vi "SRDG535.PC Set Output.vi"(0 "i ref in":refnum<vi>, 1 "inversion":bool, 2 "amplitude":dbl=1.0 min=-3.0 max=4.0 format="%.2f", 3 "offset":dbl min=-3.0 max=4.0 format="%.2f", 4 "output":u16(ring) items=["T0", "A", "B", "AB", "C", "D", "CD"], 5 "error IO":errorcluster, 7 "mode":i32(ring) items=["TTL", "NIM", "ECL", "VAR"], 9 "load":bool) -> (14 "i ref out":refnum<vi>, 19 "error out":errorcluster)   [LabVIEW 2014, in "SRDG535.lvlib"]
doc: "This VI communicates with the hardware."
uses:
  SRDG535.lvlib
  CSPhelix/PH_Common/PH_Common.lvlib
  non_GPL/instr.lib/srdg535/Stanford Research DG535 - Driver np.lvlib
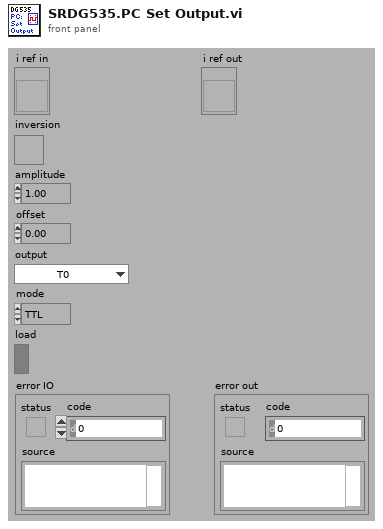
[diagram p1: front panel]
types:
  T1 = typedef "SRDG535.lvlib/SRDG535.i attribute.ctl" = cluster{"GPIB address":string, "Device error":errorcluster, "GUI Refs":cluster{"Delete":refnum<vi>, "Device Error":refnum<vi>, "Information":refnum<vi>, "Output":refnum<vi>, "Delay":refnum<vi>, "Trigger":refnum<vi>}, "Output Settings":T2, "Service ID Rate":i32, "Service IDs Channelinfo":i32[], "Delay Settings":T4, "Trigger Settings":T5}
  T2 = typedef "SRDG535.lvlib/SRDG535.Output.ctl" = cluster{"CH T0":T3, "CH A":T3, "CH B":T3, "CH AB":T3, "CH C":T3, "CH D":T3, "CH CD":T3}
  T3 = typedef "SRDG535.lvlib/SRDG535.Channel Output.ctl" = cluster{"Inversion":bool, "Amplitude (V)":dbl, "Offset (V)":dbl, "Mode":i32, "Load":bool}
  T4 = typedef "SRDG535.lvlib/SRDG535.Delay.ctl" = cluster{"CH A":cluster{"rel to":u32, "Delay (s)":dbl}, "CH B":cluster{"rel to":u32, "Delay (s)":dbl}, "CH C":cluster{"rel to":u32, "Delay (s)":dbl}, "CH D":cluster{"rel to":u32, "Delay (s)":dbl}}
  T5 = typedef "SRDG535.lvlib/SRDG535.Trigger.ctl" = cluster{"trigger":u32, "Impedance":bool, "Slope":bool, "burst count":i32, "external level (V)":sgl, "Internal/Burst Rate (Hz)":dbl, "Burst Period":i32}
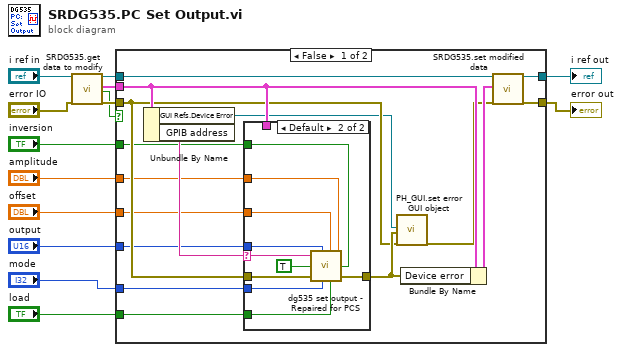
[diagram p0: block diagram]
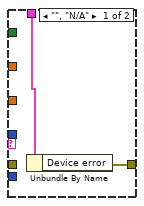
[diagram p2: hidden frame]
diagram:
  n1 = call "SRDG535.get data to modify.vi"("i ref in"="i ref in", "error in (no error)"="error IO") -> ("i ref out"=w10:refnum<vi>, "i attribute"=w14:T1, "timed out"=w7:bool, "error out"=w12:errorcluster)  [unwired: 14 in]
  n2 = case shown="False" w7 {
    tunnel: w14 -> [w30 _]
    tunnel: [w28 w43] -> w13
    tunnel: w12 -> [w22 w43]
    tunnel: [w27 w44] -> w11
    tunnel: w10 -> [w26 w44]
    tunnel: "load" -> [w20 _]
    tunnel: "mode" -> [w19 _]
    tunnel: "output" -> [w18 _]
    tunnel: "offset" -> [w17 _]
    tunnel: "amplitude" -> [w16 _]
    tunnel: "inversion" -> [w15 _]
    frame False {
      n3 = Unbundle By Name(w30) -> ("GUI Refs.Device Error"=w21:refnum<vi>, "GPIB address"=w25:string)
      n4 = case shown="Default" w25 {
        selector: w25 -> [_ w41]
        tunnel: w22 -> [_ w42]
        tunnel: [w31 w40] -> w24
        tunnel: w30 -> [w32 _]
        tunnel: w20 -> [_ w38]
        tunnel: w19 -> [_ w37]
        tunnel: w18 -> [_ w36]
        tunnel: w17 -> [_ w35]
        tunnel: w16 -> [_ w34]
        tunnel: w15 -> [_ w33]
        frame "", "N/A" {
          n5 = Unbundle By Name(w32) -> ("Device error"=w31:errorcluster)
        }
        frame Default {
          n6 = call "dg535 set output - Repaired for PCS.vi"("GPIB address"=w41, "output"=w36, "set"=TRUE, "error in"=w42, "mode"=w37, "offset"=w35, "amplitude"=w34, "inversion"=w33, "load"=w38) -> ("error out"=w40:errorcluster)
        }
      }
      n7 = call "PH_GUI.set error GUI object.vi"("GUI Refs.Device Error"=w21, "error to set"=w24, "error in (no error)"=w22) -> ("error out"=w23:errorcluster)  [unwired: 16 in]
      n8 = Bundle By Name(cluster=w30, "Device error"=w24) -> (w29:T1)
      n9 = call "SRDG535.set modified data.vi"("i ref in"=w26, "i attribute"=w29, "error in (no error)"=w23) -> ("i ref out"=w27:refnum<vi>, "error out"=w28:errorcluster)  [unwired: 15 in]
    }
    frame True {
    }
  }
  "error out" <- w13
  "i ref out" <- w11
